vi "WSVCAP SHL FPGA LL I2C Set Data Enable State.vi"(0 "State":bool, 11 "error in (no error)":errorcluster, 14 "UUT Set (0/1)":u8) -> (15 "error out":errorcluster)   [LabVIEW 2012]
uses:
  <vilib>/eio/EIOMethodNode/EIOMethodNode.xnode
  <vilib>/rvi/eio/common/nirviEmuTemplateMethod_errors.vi
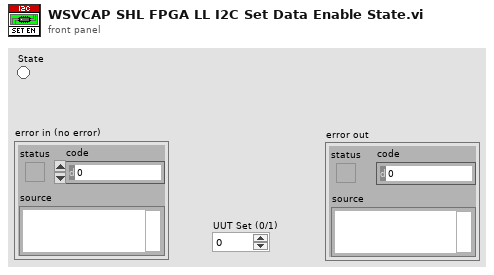
[diagram p1: front panel]
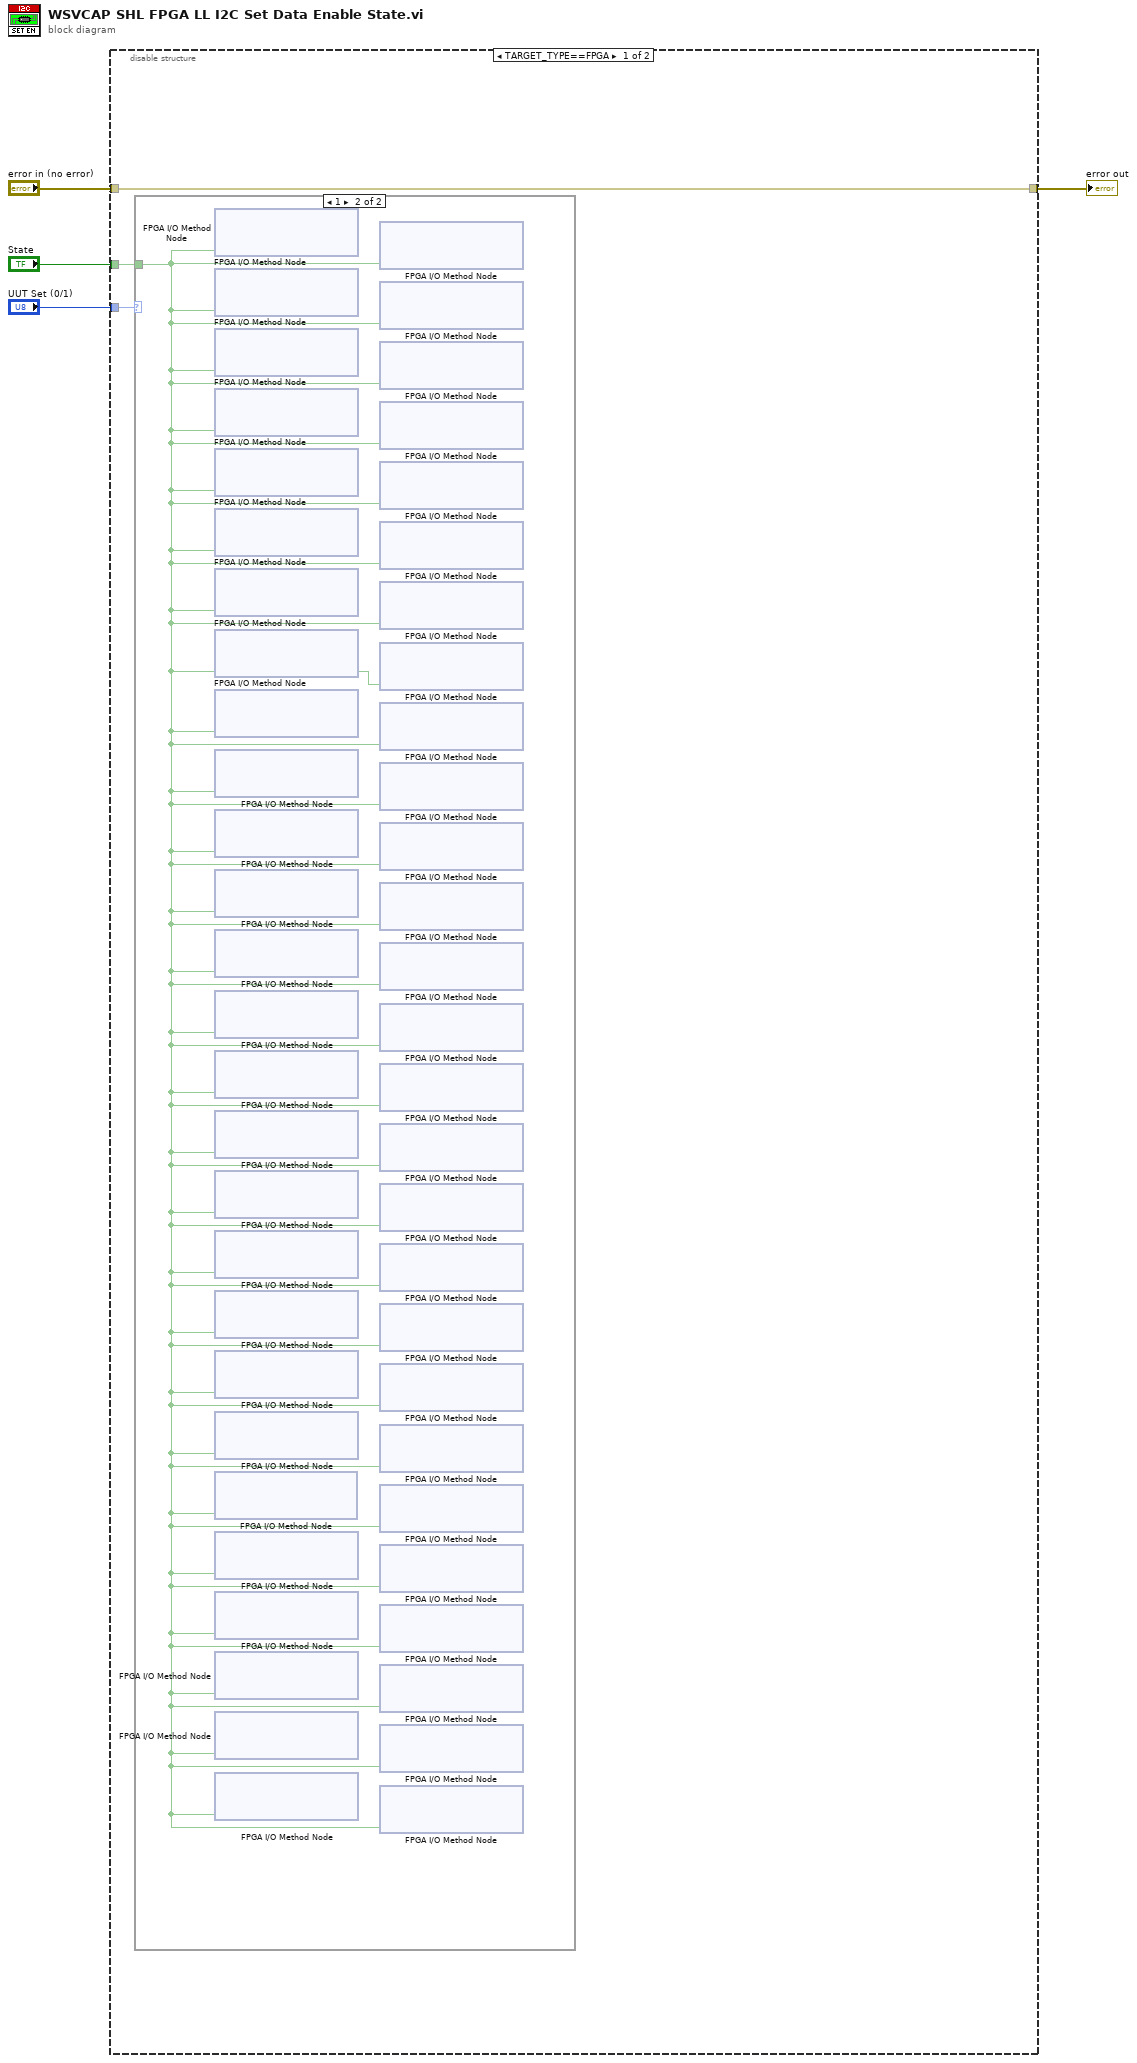
[diagram p0: block diagram]
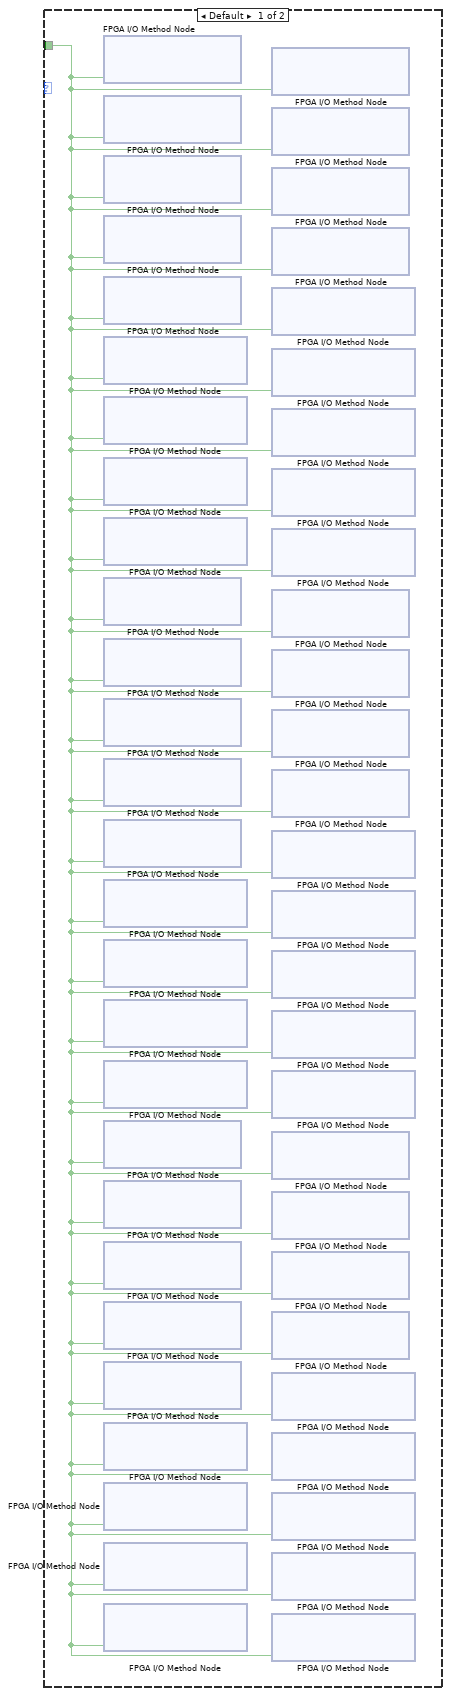
[diagram p2: hidden frame]
diagram:
  n1 = disable-structure shown="TARGET_TYPE==FPGA" {
    disable-tunnel: "State" -> [w5 _]
    disable-tunnel: [w7 w10] -> w3
    disable-tunnel: "error in (no error)" -> [w7 w10]
    disable-tunnel: "UUT Set (0/1)" -> [w6 _]
    frame condition #0 {
      n2 = case shown="1" w6 {
        tunnel: w5 -> [w8 w9]
        frame Default {
          n3 = xnode "FPGA I/O Method Node"("Enable"=w8) -> ()  [unwired: 1 in, 1 out]
          n4 = xnode "FPGA I/O Method Node"("Enable"=w8) -> ()  [unwired: 1 in, 1 out]
          n5 = xnode "FPGA I/O Method Node"("Enable"=w8) -> ()  [unwired: 1 in, 1 out]
          n6 = xnode "FPGA I/O Method Node"("Enable"=w8) -> ()  [unwired: 1 in, 1 out]
          n7 = xnode "FPGA I/O Method Node"("Enable"=w8) -> ()  [unwired: 1 in, 1 out]
          n8 = xnode "FPGA I/O Method Node"("Enable"=w8) -> ()  [unwired: 1 in, 1 out]
          n9 = xnode "FPGA I/O Method Node"("Enable"=w8) -> ()  [unwired: 1 in, 1 out]
          n10 = xnode "FPGA I/O Method Node"("Enable"=w8) -> ()  [unwired: 1 in, 1 out]
          n11 = xnode "FPGA I/O Method Node"("Enable"=w8) -> ()  [unwired: 1 in, 1 out]
          n12 = xnode "FPGA I/O Method Node"("Enable"=w8) -> ()  [unwired: 1 in, 1 out]
          n13 = xnode "FPGA I/O Method Node"("Enable"=w8) -> ()  [unwired: 1 in, 1 out]
          n14 = xnode "FPGA I/O Method Node"("Enable"=w8) -> ()  [unwired: 1 in, 1 out]
          n15 = xnode "FPGA I/O Method Node"("Enable"=w8) -> ()  [unwired: 1 in, 1 out]
          n16 = xnode "FPGA I/O Method Node"("Enable"=w8) -> ()  [unwired: 1 in, 1 out]
          n17 = xnode "FPGA I/O Method Node"("Enable"=w8) -> ()  [unwired: 1 in, 1 out]
          n18 = xnode "FPGA I/O Method Node"("Enable"=w8) -> ()  [unwired: 1 in, 1 out]
          n19 = xnode "FPGA I/O Method Node"("Enable"=w8) -> ()  [unwired: 1 in, 1 out]
          n20 = xnode "FPGA I/O Method Node"("Enable"=w8) -> ()  [unwired: 1 in, 1 out]
          n21 = xnode "FPGA I/O Method Node"("Enable"=w8) -> ()  [unwired: 1 in, 1 out]
          n22 = xnode "FPGA I/O Method Node"("Enable"=w8) -> ()  [unwired: 1 in, 1 out]
          n23 = xnode "FPGA I/O Method Node"("Enable"=w8) -> ()  [unwired: 1 in, 1 out]
          n24 = xnode "FPGA I/O Method Node"("Enable"=w8) -> ()  [unwired: 1 in, 1 out]
          n25 = xnode "FPGA I/O Method Node"("Enable"=w8) -> ()  [unwired: 1 in, 1 out]
          n26 = xnode "FPGA I/O Method Node"("Enable"=w8) -> ()  [unwired: 1 in, 1 out]
          n27 = xnode "FPGA I/O Method Node"("Enable"=w8) -> ()  [unwired: 1 in, 1 out]
          n28 = xnode "FPGA I/O Method Node"("Enable"=w8) -> ()  [unwired: 1 in, 1 out]
          n29 = xnode "FPGA I/O Method Node"("Enable"=w8) -> ()  [unwired: 1 in, 1 out]
          n30 = xnode "FPGA I/O Method Node"("Enable"=w8) -> ()  [unwired: 1 in, 1 out]
          n31 = xnode "FPGA I/O Method Node"("Enable"=w8) -> ()  [unwired: 1 in, 1 out]
          n32 = xnode "FPGA I/O Method Node"("Enable"=w8) -> ()  [unwired: 1 in, 1 out]
          n33 = xnode "FPGA I/O Method Node"("Enable"=w8) -> ()  [unwired: 1 in, 1 out]
          n34 = xnode "FPGA I/O Method Node"("Enable"=w8) -> ()  [unwired: 1 in, 1 out]
          n35 = xnode "FPGA I/O Method Node"("Enable"=w8) -> ()  [unwired: 1 in, 1 out]
          n36 = xnode "FPGA I/O Method Node"("Enable"=w8) -> ()  [unwired: 1 in, 1 out]
          n37 = xnode "FPGA I/O Method Node"("Enable"=w8) -> ()  [unwired: 1 in, 1 out]
          n38 = xnode "FPGA I/O Method Node"("Enable"=w8) -> ()  [unwired: 1 in, 1 out]
          n39 = xnode "FPGA I/O Method Node"("Enable"=w8) -> ()  [unwired: 1 in, 1 out]
          n40 = xnode "FPGA I/O Method Node"("Enable"=w8) -> ()  [unwired: 1 in, 1 out]
          n41 = xnode "FPGA I/O Method Node"("Enable"=w8) -> ()  [unwired: 1 in, 1 out]
          n42 = xnode "FPGA I/O Method Node"("Enable"=w8) -> ()  [unwired: 1 in, 1 out]
          n43 = xnode "FPGA I/O Method Node"("Enable"=w8) -> ()  [unwired: 1 in, 1 out]
          n44 = xnode "FPGA I/O Method Node"("Enable"=w8) -> ()  [unwired: 1 in, 1 out]
          n45 = xnode "FPGA I/O Method Node"("Enable"=w8) -> ()  [unwired: 1 in, 1 out]
          n46 = xnode "FPGA I/O Method Node"("Enable"=w8) -> ()  [unwired: 1 in, 1 out]
          n47 = xnode "FPGA I/O Method Node"("Enable"=w8) -> ()  [unwired: 1 in, 1 out]
          n48 = xnode "FPGA I/O Method Node"("Enable"=w8) -> ()  [unwired: 1 in, 1 out]
          n49 = xnode "FPGA I/O Method Node"("Enable"=w8) -> ()  [unwired: 1 in, 1 out]
          n50 = xnode "FPGA I/O Method Node"("Enable"=w8) -> ()  [unwired: 1 in, 1 out]
          n51 = xnode "FPGA I/O Method Node"("Enable"=w8) -> ()  [unwired: 1 in, 1 out]
          n52 = xnode "FPGA I/O Method Node"("Enable"=w8) -> ()  [unwired: 1 in, 1 out]
          n53 = xnode "FPGA I/O Method Node"("Enable"=w8) -> ()  [unwired: 1 in, 1 out]
          n54 = xnode "FPGA I/O Method Node"("Enable"=w8) -> ()  [unwired: 1 in, 1 out]
          n55 = xnode "FPGA I/O Method Node"("Enable"=w8) -> ()  [unwired: 1 in, 1 out]
          n56 = xnode "FPGA I/O Method Node"("Enable"=w8) -> ()  [unwired: 1 in, 1 out]
        }
        frame 1 {
          n57 = xnode "FPGA I/O Method Node"("Enable"=w9) -> ()  [unwired: 1 in, 1 out]
          n58 = xnode "FPGA I/O Method Node"("Enable"=w9) -> ()  [unwired: 1 in, 1 out]
          n59 = xnode "FPGA I/O Method Node"("Enable"=w9) -> ()  [unwired: 1 in, 1 out]
          n60 = xnode "FPGA I/O Method Node"("Enable"=w9) -> ()  [unwired: 1 in, 1 out]
          n61 = xnode "FPGA I/O Method Node"("Enable"=w9) -> ()  [unwired: 1 in, 1 out]
          n62 = xnode "FPGA I/O Method Node"("Enable"=w9) -> ()  [unwired: 1 in, 1 out]
          n63 = xnode "FPGA I/O Method Node"("Enable"=w9) -> ()  [unwired: 1 in, 1 out]
          n64 = xnode "FPGA I/O Method Node"("Enable"=w9) -> ()  [unwired: 1 in, 1 out]
          n65 = xnode "FPGA I/O Method Node"("Enable"=w9) -> ()  [unwired: 1 in, 1 out]
          n66 = xnode "FPGA I/O Method Node"("Enable"=w9) -> ()  [unwired: 1 in, 1 out]
          n67 = xnode "FPGA I/O Method Node"("Enable"=w9) -> ()  [unwired: 1 in, 1 out]
          n68 = xnode "FPGA I/O Method Node"("Enable"=w9) -> ()  [unwired: 1 in, 1 out]
          n69 = xnode "FPGA I/O Method Node"("Enable"=w9) -> ()  [unwired: 1 in, 1 out]
          n70 = xnode "FPGA I/O Method Node"("Enable"=w9) -> ()  [unwired: 1 in, 1 out]
          n71 = xnode "FPGA I/O Method Node"("Enable"=w9) -> ()  [unwired: 1 in, 1 out]
          n72 = xnode "FPGA I/O Method Node"("Enable"=w9) -> ()  [unwired: 1 in, 1 out]
          n73 = xnode "FPGA I/O Method Node"("Enable"=w9) -> ()  [unwired: 1 in, 1 out]
          n74 = xnode "FPGA I/O Method Node"("Enable"=w9) -> ()  [unwired: 1 in, 1 out]
          n75 = xnode "FPGA I/O Method Node"("Enable"=w9) -> ()  [unwired: 1 in, 1 out]
          n76 = xnode "FPGA I/O Method Node"("Enable"=w9) -> ()  [unwired: 1 in, 1 out]
          n77 = xnode "FPGA I/O Method Node"("Enable"=w9) -> ()  [unwired: 1 in, 1 out]
          n78 = xnode "FPGA I/O Method Node"("Enable"=w9) -> ()  [unwired: 1 in, 1 out]
          n79 = xnode "FPGA I/O Method Node"("Enable"=w9) -> ()  [unwired: 1 in, 1 out]
          n80 = xnode "FPGA I/O Method Node"("Enable"=w9) -> ()  [unwired: 1 in, 1 out]
          n81 = xnode "FPGA I/O Method Node"("Enable"=w9) -> ()  [unwired: 1 in, 1 out]
          n82 = xnode "FPGA I/O Method Node"("Enable"=w9) -> ()  [unwired: 1 in, 1 out]
          n83 = xnode "FPGA I/O Method Node"("Enable"=w9) -> ()  [unwired: 1 in, 1 out]
          n84 = xnode "FPGA I/O Method Node"("Enable"=w9) -> ()  [unwired: 1 in, 1 out]
          n85 = xnode "FPGA I/O Method Node"("Enable"=w9) -> ()  [unwired: 1 in, 1 out]
          n86 = xnode "FPGA I/O Method Node"("Enable"=w9) -> ()  [unwired: 1 in, 1 out]
          n87 = xnode "FPGA I/O Method Node"("Enable"=w9) -> ()  [unwired: 1 in, 1 out]
          n88 = xnode "FPGA I/O Method Node"("Enable"=w9) -> ()  [unwired: 1 in, 1 out]
          n89 = xnode "FPGA I/O Method Node"("Enable"=w9) -> ()  [unwired: 1 in, 1 out]
          n90 = xnode "FPGA I/O Method Node"("Enable"=w9) -> ()  [unwired: 1 in, 1 out]
          n91 = xnode "FPGA I/O Method Node"("Enable"=w9) -> ()  [unwired: 1 in, 1 out]
          n92 = xnode "FPGA I/O Method Node"("Enable"=w9) -> ()  [unwired: 1 in, 1 out]
          n93 = xnode "FPGA I/O Method Node"("Enable"=w9) -> ()  [unwired: 1 in, 1 out]
          n94 = xnode "FPGA I/O Method Node"("Enable"=w9) -> ()  [unwired: 1 in, 1 out]
          n95 = xnode "FPGA I/O Method Node"("Enable"=w9) -> ()  [unwired: 1 in, 1 out]
          n96 = xnode "FPGA I/O Method Node"("Enable"=w9) -> ()  [unwired: 1 in, 1 out]
          n97 = xnode "FPGA I/O Method Node"("Enable"=w9) -> ()  [unwired: 1 in, 1 out]
          n98 = xnode "FPGA I/O Method Node"("Enable"=w9) -> ()  [unwired: 1 in, 1 out]
          n99 = xnode "FPGA I/O Method Node"("Enable"=w9) -> ()  [unwired: 1 in, 1 out]
          n100 = xnode "FPGA I/O Method Node"("Enable"=w9) -> ()  [unwired: 1 in, 1 out]
          n101 = xnode "FPGA I/O Method Node"("Enable"=w9) -> ()  [unwired: 1 in, 1 out]
          n102 = xnode "FPGA I/O Method Node"("Enable"=w9) -> ()  [unwired: 1 in, 1 out]
          n103 = xnode "FPGA I/O Method Node"("Enable"=w9) -> ()  [unwired: 1 in, 1 out]
          n104 = xnode "FPGA I/O Method Node"("Enable"=w9) -> ()  [unwired: 1 in, 1 out]
          n105 = xnode "FPGA I/O Method Node"("Enable"=w9) -> ()  [unwired: 1 in, 1 out]
          n106 = xnode "FPGA I/O Method Node"("Enable"=w9) -> ()  [unwired: 1 in, 1 out]
          n107 = xnode "FPGA I/O Method Node"("Enable"=w9) -> ()  [unwired: 1 in, 1 out]
          n108 = xnode "FPGA I/O Method Node"("Enable"=w9) -> ()  [unwired: 1 in, 1 out]
          n109 = xnode "FPGA I/O Method Node"("Enable"=w9) -> ()  [unwired: 1 in, 1 out]
          n110 = xnode "FPGA I/O Method Node"("Enable"=w9) -> ()  [unwired: 1 in, 1 out]
        }
      }
    }
    frame condition #1 (active) {
    }
  }
  "error out" <- w3
